vi "VI Quality.vi"() -> ()   [LabVIEW 2018, in "VI Quality.lvlib"]
doc: "This is the top level VI for the VI Quality Assurance user interface."
uses:
  VI Quality.lvlib
  <vilib>/LabVIEW Icon API/LabVIEW Icon API.lvlib
  <vilib>/Utility/miscctls.llb/LVRowAndColumnUnsignedTypeDef.ctl
  <vilib>/Utility/miscctls.llb/LVPointTypeDef.ctl
  <vilib>/Utility/miscctls.llb/LVSelectionTypeDef.ctl
  <vilib>/LabVIEW Icon API/lv_icon/Classes/Icon/Icon.lvclass
  Controls/VIQA VI Info.ctl
  Controls/VIQA Audit Ignore.ctl
panel:
  in  "Fix All":bool
  in  "ResetVI":bool
  out "VIBusy":bool
  in  "Edit Icon":bool
  in  "Reset Legal":bool
  in  "Legal":string caption="Legal Marking"
  out "VI Name":string
  in  "Ignore":T1
  in  "Abort":bool
  out "BusyAud":bool
  out "AuditSlide":dbl(slide) scale=0.0..100.0
  in  "AuditMCLB":i32(listbox) caption="Audit"
  in  "Audit":bool
  out "Busy":bool
  in  "Filter":enum16{"None", "No Description"}(ring)
  in  "Path Refresh":bool
  in  "Apply":bool
  in  "VI Description":string
  out "VI Path":path
  in  "Stop":bool
  out "ConPane":picture caption="VI Icon"
  in  "Project Tree":string[](tree)
  in  "Path":path caption="Path (*.lvproj)"
  # "Audit"
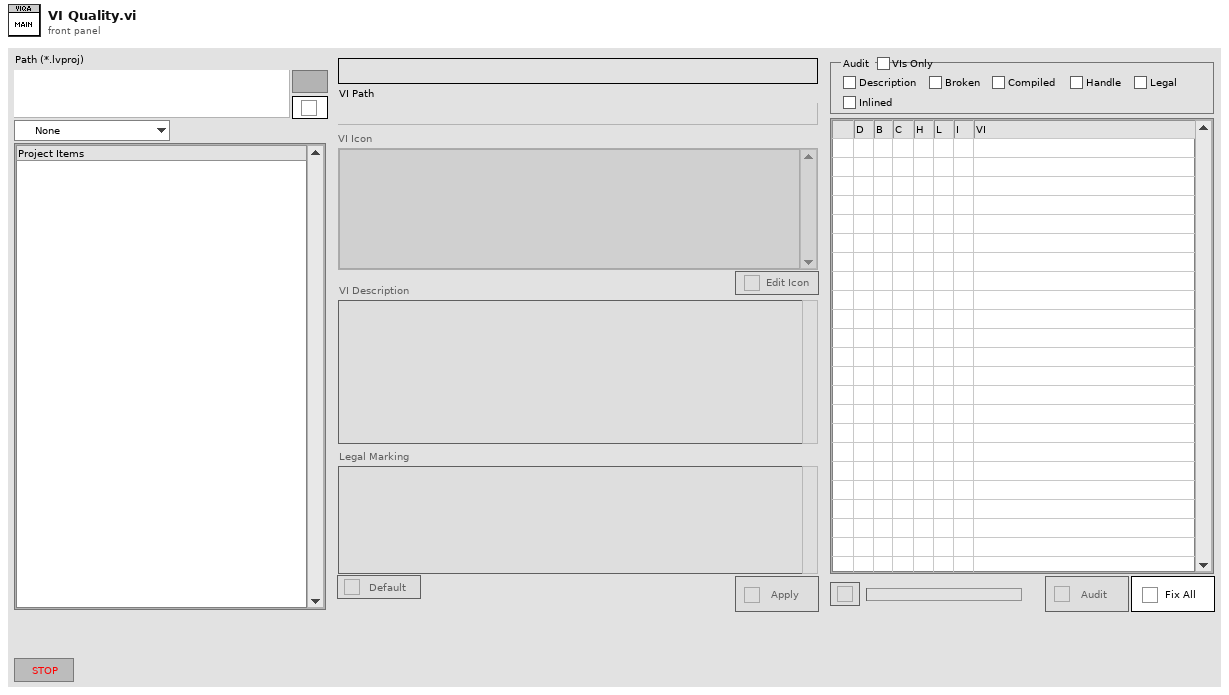
[diagram p1: front panel]
types:
  T1 = cluster{"Controls":bool, "Description":bool, "Broken":bool, "Compiled":bool, "Handle":bool, "Legal":bool, "Inlined":bool}
  T2 = cluster{"image type":i32, "image depth":i32, "image":u8[], "mask":u8[], "colors":u32[], "Rectangle":cluster{"left":i16, "top":i16, "right":i16, "bottom":i16}}[]
  T3 = typedef "VI Quality.lvlib/VIQA VI Info.ctl" = cluster{"Path":path, "Desc":string, "ConPane":cluster{"image type":i32, "image depth":i32, "image":u8[], "mask":u8[], "colors":u32[], "Rectangle":cluster{"left":i16, "top":i16, "right":i16, "bottom":i16}}, "Legal":string, "Icon":refnum<class "Icon.lvclass">, "VIType":enum32{"invalid VI type", "Standard VI", "Control VI", "Global VI", "Polymorphic VI", "Configuration VI", "SubSystem", "Facade VI", "Method VI", "Statechart Diagram VI"}, "ItemID":string}
  T4 = cluster{"Project Tree":refnum<vi>, "App Ref":refnum<vi>, "Project":refnum<vi>, "My Computer":refnum<vi>, "VI Refnum":refnum<vi>, "VI Info":T3, "AuditMCLB":refnum<vi>, "AuditSlide":refnum<vi>, "NewDesc":string, "NewLegal":string, "NewIcon":bool, "Abort":refnum<vi>}
  T5 = typedef "LVRowAndColumnUnsignedTypeDef.ctl" = cluster{"Row":u32, "Column":u32}
  T6 = typedef "VI Quality.lvlib/VIQA Audit Ignore.ctl" = cluster{"Controls":bool, "Description":bool, "Broken":bool, "Compiled":bool, "Handle":bool, "Legal":bool, "Inline":bool}
  T7 = typedef "LVPointTypeDef.ctl" = cluster{"Horizontal":i16, "Vertical":i16}
  T8 = typedef "LVSelectionTypeDef.ctl" = cluster{"Selection Start":u32, "Selection End":u32}
  T9 = cluster{"image type":i32, "image depth":i32, "image":u8[], "mask":u8[], "colors":u32[], "Rectangle":cluster{"left":i16, "top":i16, "right":i16, "bottom":i16}}
  T10 = enum32{"invalid VI type", "Standard VI", "Control VI", "Global VI", "Polymorphic VI", "Configuration VI", "SubSystem", "Facade VI", "Method VI", "Statechart Diagram VI"}
  T11 = enum8{"Enabled", "Disabled", "Disabled and Grayed Out"}
  T12 = typedef "imagedata.ctl" = cluster{"image type":i32, "image depth":i32, "image":u8[], "mask":u8[], "colors":u32[], "Rectangle":cluster{"left":i16, "top":i16, "right":i16, "bottom":i16}}
  T13 = cluster{"Shift":bool, "Ctrl":bool, "Alt":bool, "Cmd":bool, "Opt":bool}
  T14 = typedef "eventvkey.ctl" = enum16{"ASCII", "Enter", "Return", "Shift", "Ctrl", "Alt", "Cmd", "Opt", "Caps", "NumLock", "Clear", "Break", "Up", "Down", "Left", "Right", "Insert", "Delete", "Home", "End", "PageUp", "PageDown", "Escape", "Help", "Pause", "ScrollLock", "F1", "F2", "F3", "F4", "F5", "F6", "F7", "F8", "F9", "F10", "F11", "F12", "F13", "F14", "F15", "F16", "F17", "F18", "F19", "F20", "F21", "F22", "F23", "F24", "Play", "VolumeUp", "VolumeDown", "Mute", "Two Byte Char"}
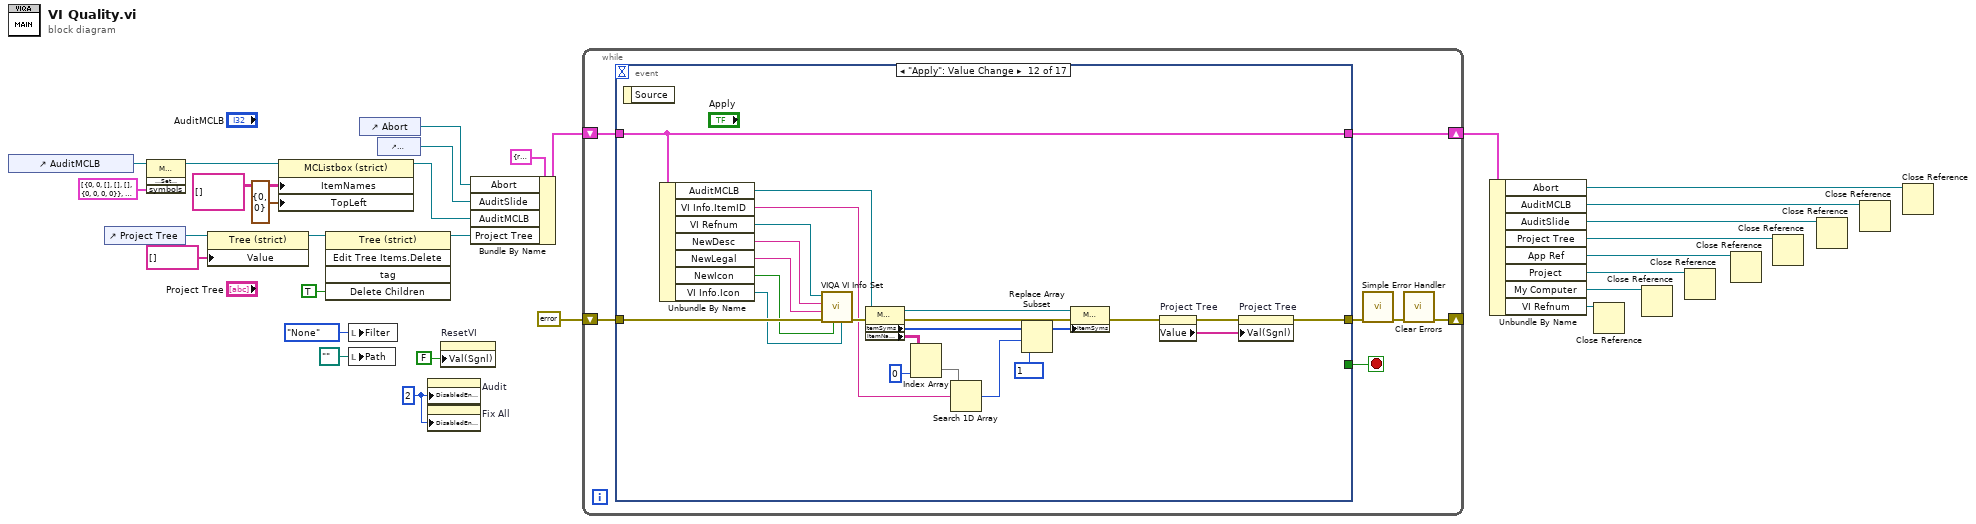
[diagram p0: block diagram]
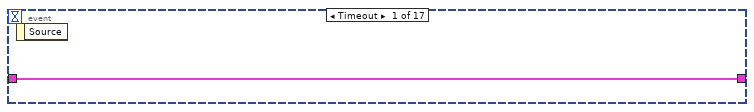
[diagram p2: hidden frame]
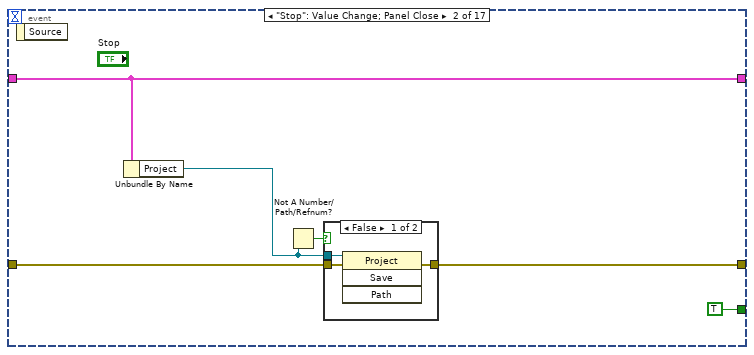
[diagram p3: hidden frame]
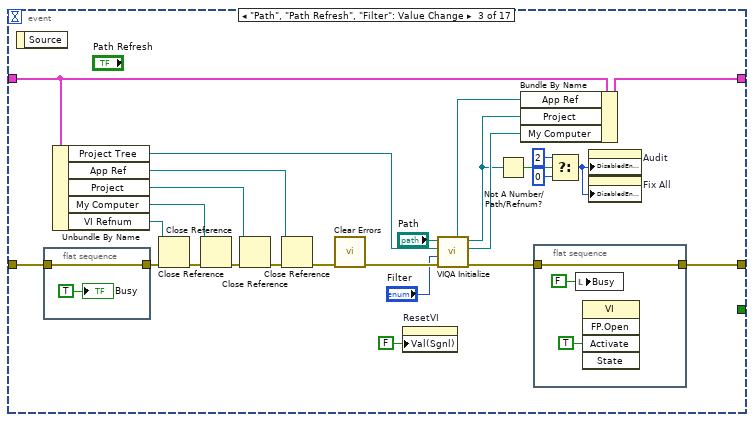
[diagram p5: hidden frame]
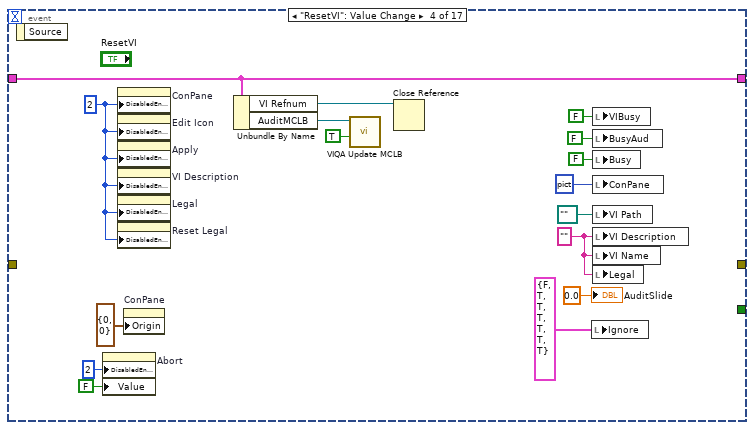
[diagram p6: hidden frame]
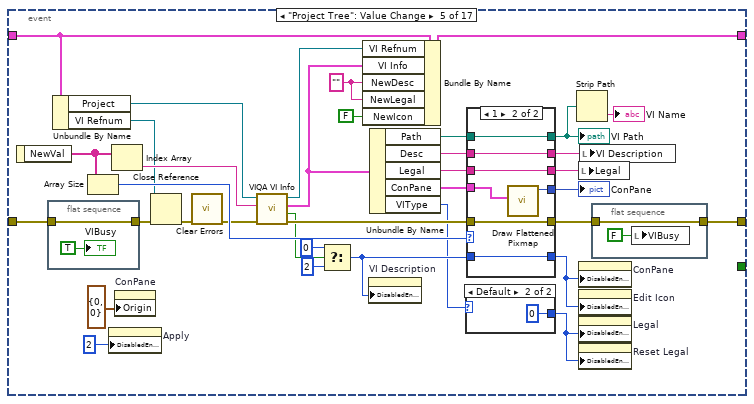
[diagram p7: hidden frame]
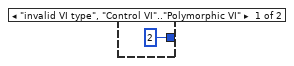
[diagram p8: hidden frame]
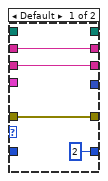
[diagram p9: hidden frame]
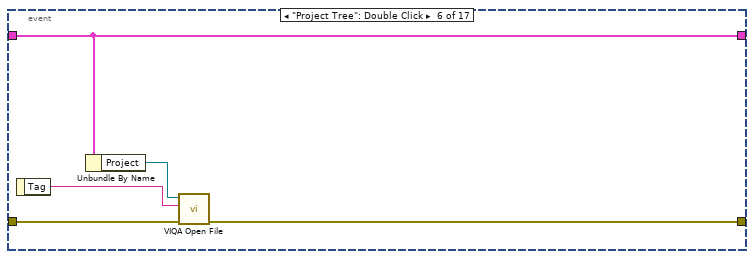
[diagram p10: hidden frame]
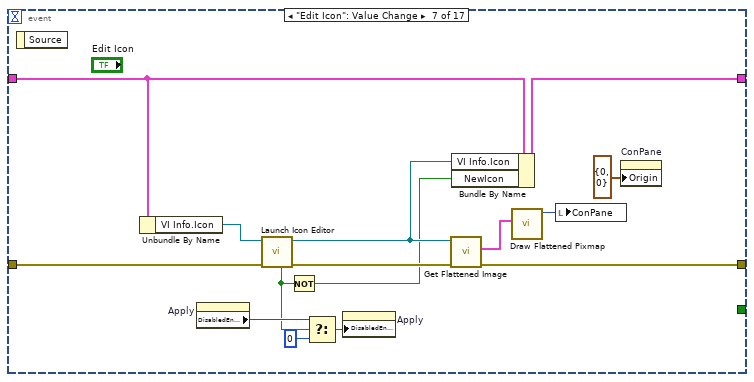
[diagram p11: hidden frame]
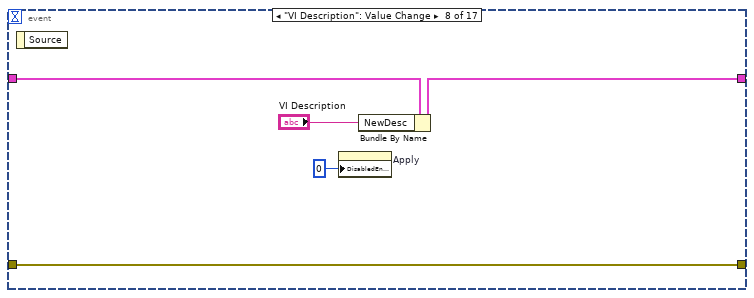
[diagram p12: hidden frame]
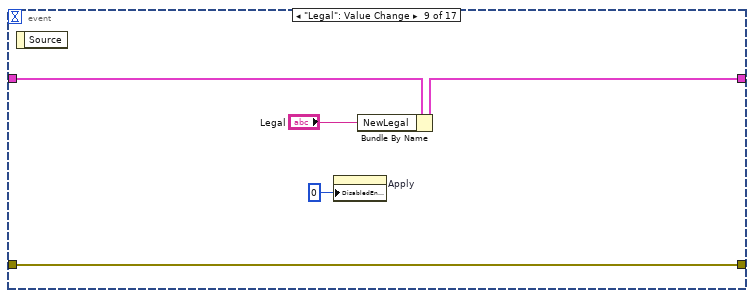
[diagram p13: hidden frame]
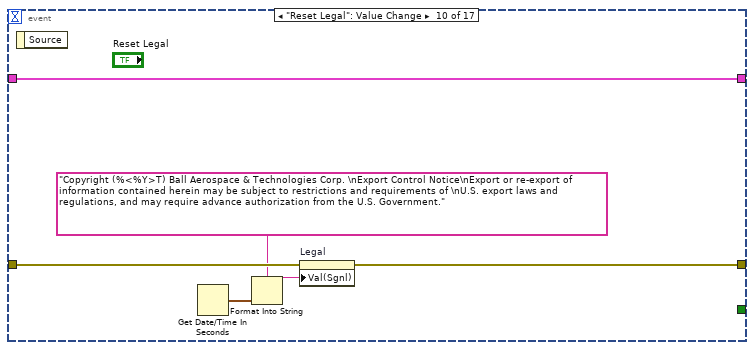
[diagram p14: hidden frame]
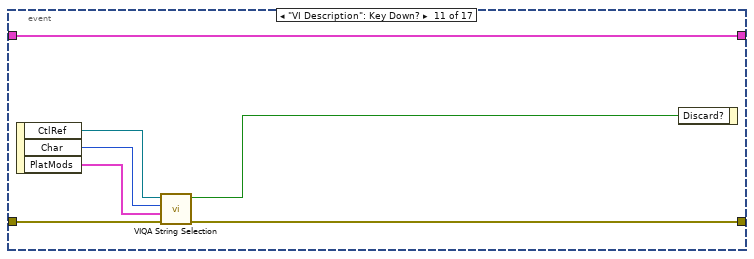
[diagram p15: hidden frame]
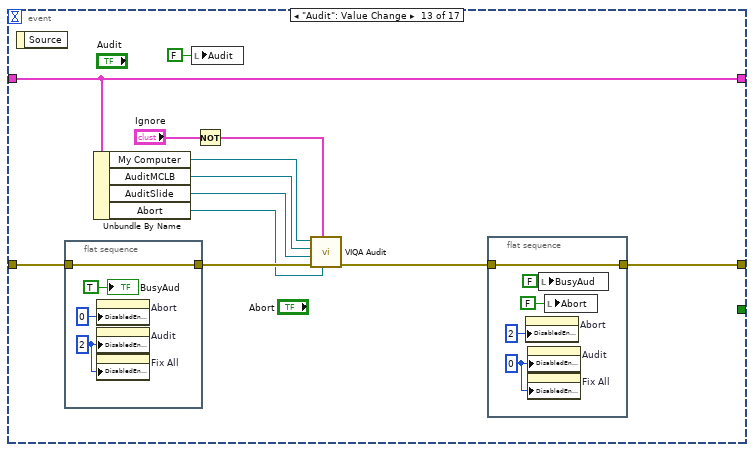
[diagram p16: hidden frame]
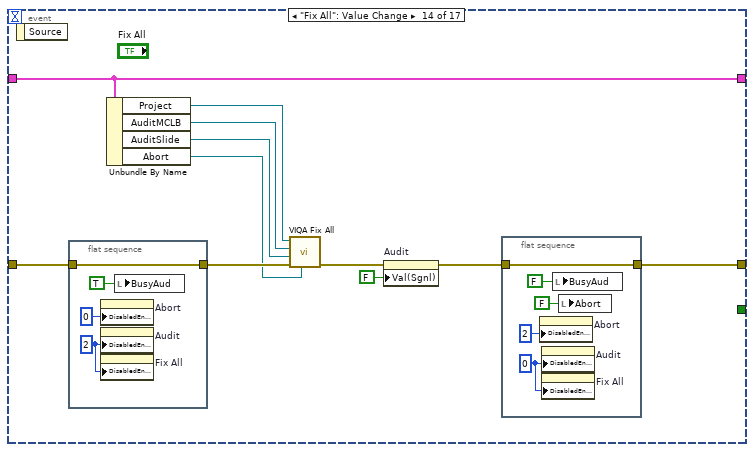
[diagram p17: hidden frame]
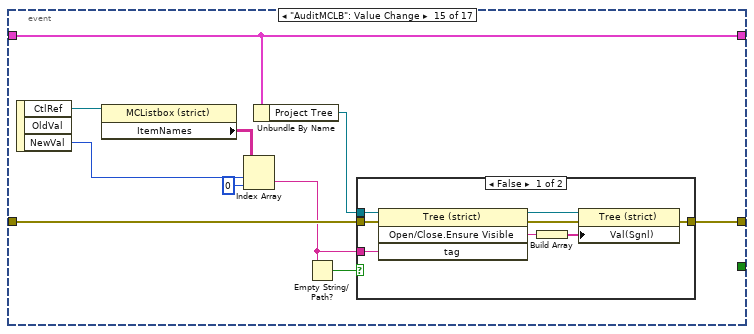
[diagram p18: hidden frame]
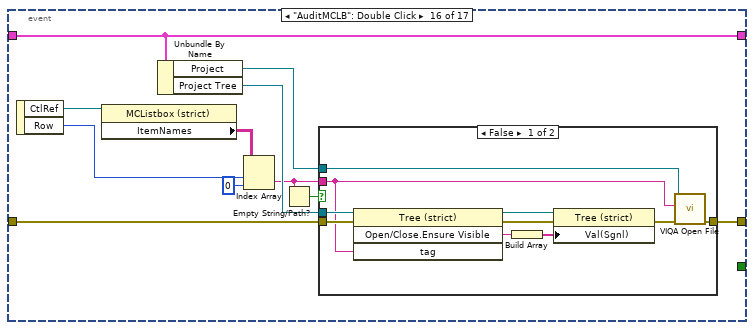
[diagram p20: hidden frame]
diagram:
  w5 = u8 2
  n1 = control-ref of="AuditMCLB"() -> (w15:refnum<vi>)
  n2 = control-ref of="Project Tree"() -> (w26:refnum<vi>)
  n3 = invoke class="MCListbox (strict)" method="Custom Item Symbols.Set Symbol Array"(reference=w15, "symbols"=T2 [{"image type"=0, "image depth"=0, "image"=[], "mask"=[], "colors"=[], "Rectangle"={"left"=0, "top"=0, "right"=0, "bottom"=0}}, {"image type"=0, "image depth"=32, "image"=[0, 0, 0, 0, 0, 0, 0, 0, 0, 0, 0, 0, 0, 0, 0, 0, 0, 0, 0, 0, 0, 0, 0, 0, 0, 0, 0, 0, 0, 0, 0, 0, 0, 0, 0, 0, 0, 0, 0, 0, 0, 0, 0, 0, 0, 0, 0, 0, 0, 0, 0, 0, 0, 0, 0, 0, 0, 0, 0, 0, 0, 0, 0, 0, 0, 0, 0, 0, 0, 0, 0, 0, 0, 0, 0, 0, 0, 0, 0, 0, 0, 0, 0, 0, 0, 0, 0, 0, 0, 0, 0, 0, 0, 0, 0, 0, 0, 0, 0, 0, 0, 0, 0, 0, 0, 0, 0, 0, 0, 0, 0, 0, 0, 0, 0, 0, 0, 0, 0, 0, 0, 0, 0, 0, 0, 0, 0, 0, 0, 0, 0, 0, 0, 0, 0, 0, 0, 0, 0, 0, 0, 0, 0, 0, 0, 0, 0, 0, 0, 0, 0, 0, 0, 0, 0, 0, 0, 0, 0, 0, 0, 0, 0, 0, 0, 0, 0, 0, 0, 0, 0, 0, 0, 0, 0, 0, 0, 0, 0, 0, 0, 0, 0, 0, 255, 133, 241, 88, 255, 85, 205, 56, 0, 0, 0, 0, 0, 0, 0, 0, 0, 0, 0, 0, 0, 0, 0, 0, 0, 0, 0, 0, 0, 0, 0, 0, 0, 0, 0, 0, 0, 0, 0, 0, 0, 0, 0, 0, 0, 0, 0, 0, 0, 0, 0, 0, 0, 0, 0, 0, 255, 121, 232, 80, 255, 121, 232, 80, 255, 121, 232, 80, 255, 85, 205, 56, 0, 0, 0, 0, 0, 0, 0, 0, 0, 0, 0, 0, 0, 0, 0, 0, 0, 0, 0, 0, 0, 0, 0, 0, 0, 0, 0, 0, 0, 0, 0, 0, 0, 0, 0, 0, 0, 0, 0, 0, 0, 0, 0, 0, 255, 109, 223, 72, 255, 109, 223, 72, 255, 109, 223, 72, 255, 109, 223, 72, 255, 0, 141, 0, 0, 0, 0, 0, 0, 0, 0, 0, 0, 0, 0, 0, 0, 0, 0, 0, 0, 0, 0, 0, 0, 0, 0, 0, 0, 0, 0, 0, 0, 0, 0, 0, 0, 0, 0, 0, 0, 0, 0, 0, 255, 97, 214, 64, 255, 97, 214, 64, 255, 97, 214, 64, 255, 97, 214, 64, 255, 0, 141, 0, 0, 0, 0, 0, 0, 0, 0, 0, 0, 0, 0, 0, 0, 0, 0, 0, 0, 0, 0, 0, 0, 0, 0, 0, 0, 0, 0, 0, 0, 0, 0, 0, 0, 0, 0, 0, 0, 0, 0, 0, 255, 85, 205, 56, 255, 85, 205, 56, 255, 85, 205, 56, 255, 85, 205, 56, 255, 0, 141, 0, 0, 0, 0, 0, 0, 0, 0, 0, 0, 0, 0, 0, 255, 73, 196, 48, 255, 73, 196, 48, 255, 73, 196, 48, 0, 0, 0, 0, 0, 0, 0, 0, 0, 0, 0, 0, 0, 0, 0, 0, 255, 73, 196, 48, 255, 73, 196, 48, 255, 73, 196, 48, 255, 73, 196, 48, 255, 0, 141, 0, 0, 0, 0, 0, 0, 0, 0, 0, 0, 0, 0, 0, 0, 0, 0, 0, 255, 12, 150, 8, 255, 60, 186, 40, 255, 60, 186, 40, 255, 60, 186, 40, 0, 0, 0, 0, 0, 0, 0, 0, 255, 60, 186, 40, 255, 60, 186, 40, 255, 60, 186, 40, 255, 60, 186, 40, 255, 0, 141, 0, 0, 0, 0, 0, 0, 0, 0, 0, 0, 0, 0, 0, 0, 0, 0, 0, 0, 0, 0, 0, 255, 0, 141, 0, 255, 48, 177, 32, 255, 48, 177, 32, 255, 48, 177, 32, 255, 48, 177, 32, 255, 48, 177, 32, 255, 48, 177, 32, 255, 48, 177, 32, 255, 48, 177, 32, 255, 0, 141, 0, 0, 0, 0, 0, 0, 0, 0, 0, 0, 0, 0, 0, 0, 0, 0, 0, 0, 0, 0, 0, 0, 0, 0, 0, 0, 0, 0, 0, 255, 0, 141, 0, 255, 36, 168, 24, 255, 36, 168, 24, 255, 36, 168, 24, 255, 36, 168, 24, 255, 36, 168, 24, 255, 36, 168, 24, 255, 0, 141, 0, 0, 0, 0, 0, 0, 0, 0, 0, 0, 0, 0, 0, 0, 0, 0, 0, 0, 0, 0, 0, 0, 0, 0, 0, 0, 0, 0, 0, 0, 0, 0, 0, 0, 0, 0, 0, 255, 0, 141, 0, 255, 24, 159, 16, 255, 24, 159, 16, 255, 24, 159, 16, 255, 24, 159, 16, 255, 0, 141, 0, 0, 0, 0, 0, 0, 0, 0, 0, 0, 0, 0, 0, 0, 0, 0, 0, 0, 0, 0, 0, 0, 0, 0, 0, 0, 0, 0, 0, 0, 0, 0, 0, 0, 0, 0, 0, 0, 0, 0, 0, 0, 0, 0, 0, 255, 0, 141, 0, 255, 12, 150, 8, 255, 12, 150, 8, 255, 0, 141, 0, 0, 0, 0, 0, 0, 0, 0, 0, 0, 0, 0, 0, 0, 0, 0, 0, 0, 0, 0, 0, 0, 0, 0, 0, 0, 0, 0, 0, 0, 0, 0, 0, 0, 0, 0, 0, 0, 0, 0, 0, 0, 0, 0, 0, 0, 0, 0, 0, 0, 0, 0, 0, 255, 0, 141, 0, 255, 0, 141, 0, 0, 0, 0, 0, 0, 0, 0, 0, 0, 0, 0, 0, 0, 0, 0, 0, 0, 0, 0, 0, 0, 0, 0, 0, 0, 0, 0, 0, 0, 0, 0, 0, 0, 0, 0, 0, 0, 0, 0, 0, 0, 0, 0, 0, 0, 0, 0, 0, 0, 0, 0, 0, 0, 0, 0, 0, 0, 0, 0, 0, 0, 0, 0, 0, 0, 0, 0, 0, 0, 0, 0, 0, 0, 0, 0, 0, 0, 0, 0, 0, 0, 0, 0, 0, 0, 0, 0, 0, 0, 0, 0, 0, 0, 0, 0, 0, 0, 0, 0, 0, 0, 0, 0, 0, 0, 0, 0, 0, 0, 0, 0, 0, 0, 0, 0, 0, 0, 0, 0, 0, 0, 0, 0, 0, 0, 0, 0, 0, 0, 0, 0, 0, 0, 0, 0, 0, 0, 0, 0, 0, 0, 0, 0, 0, 0, 0, 0, 0, 0, 0, 0, 0, 0, 0, 0, 0, 0, 0, 0, 0, 0, 0, 0, 0], "mask"=[0, 0, 0, 0, 0, 3, 0, 15, 0, 31, 0, 62, 0, 124, 112, 248, 121, 240, 127, 224, 63, 192, 31, 128, 15, 0, 6, 0, 0, 0, 0, 0], "colors"=[], "Rectangle"={"left"=0, "top"=0, "right"=16, "bottom"=16}}] ("Symbols")) -> (reference out=w2:refnum<vi>)  [unwired: 2 in, 3 out]
  n4 = property class="Tree (strict)"(reference=w26, "Value"=string[] []) -> (reference out=w18:refnum<vi>)  [unwired: 1 in, 1 out]
  n5 = property class="MCListbox (strict)"(reference=w2, "ItemNames"=string[][] [] ("Item Names"), "TopLeft"=T5 {"Row"=0, "Column"=0} ("Top Left Visible Cell")) -> (reference out=w13:refnum<vi>)  [unwired: 1 in, 1 out]
  n6 = invoke class="Tree (strict)" method="Edit Tree Items.Delete"(reference=w18, "Delete Children"=TRUE ("Delete Children?")) -> (reference out=w25:refnum<vi>)  [unwired: 3 in, 4 out]
  n7 = local write "Filter"(enum16{"None", "No Description", "No Legend"}."None" ("Filter")) -> ()
  n8 = local write "Path"(path "" ("Path")) -> ()
  n9 = control-ref of="Abort"() -> (w4:refnum<vi>)
  n10 = control-ref of="AuditSlide"() -> (w14:refnum<vi>)
  n11 = property on="Audit" class="Bool (strict)"("DisabledEnum"=w5) -> ()  [unwired: 2 in, 2 out]
  n12 = property on="Fix All" class="Bool"("DisabledEnum"=w5) -> ()  [unwired: 2 in, 2 out]
  n13 = property on="ResetVI" class="Bool (strict)"("Val(Sgnl)"=FALSE ("Value (Signaling)")) -> ()  [unwired: 2 in, 2 out]
  n14 = Bundle By Name(cluster=T4 {"Project Tree"=refnum, "App Ref"=refnum, "Project"=refnum, "My Computer"=refnum, "VI Refnum"=refnum, "VI Info"={"Path"=path "", "Desc"="", "ConPane"={"image type"=0, "image depth"=0, "image"=[], "mask"=[], "colors"=[], "Rectangle"={"left"=0, "top"=0, "right"=0, "bottom"=0}}, "Legal"="", "Icon"=refnum, "VIType"=enum."invalid VI type", "ItemID"=""}, "AuditMCLB"=refnum, "AuditSlide"=refnum, "NewDesc"="", "NewLegal"="", "NewIcon"=FALSE, "Abort"=refnum} ("StateData"), "Abort"=w4, "AuditSlide"=w14, "AuditMCLB"=w13, "Project Tree"=w25) -> (w27:T4)
  n15 = while {
    shift-right: [w30] -> _
    shift-left: errorcluster {"status"=FALSE, "code"=0, "source"=""} ("error in (no error)") -> [w35]
    shift-right: [w32] -> w23
    shift-left: w27 -> [w33]
    stop <- w36 stop-if-true
    n16 = event shown="[11] \"Apply\": Value Change" {
      selector: _ -> [_ _ _ _ _ _ _ _ _ _ _ _ _ _ _ _ _]
      dyn-events: _ -> [_ _ _ _ _ _ _ _ _ _ _ _ _ _ _ _ _]
      timeout: _ -> [_ _ _ _ _ _ _ _ _ _ _ _ _ _ _ _ _]
      tunnel: [_ TRUE _ _ _ _ _ _ _ _ _ _ _ _ _ _ _] -> w36
      tunnel: w35 -> [_ w42 w56 _ w97 w152 w164 w169 w174 w182 w188 w212 w221 w241 w259 w278 w298]
      tunnel: [_ w41 w55 _ w96 w149 w161 w169 w174 w181 w187 w205 w220 w242 w258 w277 w299] -> w34
      tunnel: w33 -> [w37 w40 w72 w82 w130 w151 w167 w172 w177 w183 w190 w213 w225 w245 w261 w280 w302]
      tunnel: [w37 w40 w65 w82 w127 w151 w166 w171 w176 w183 w190 w213 w225 w245 w261 w280 w302] -> w32
      event Timeout {
        n17 = event-data() -> ()  [unwired: 1 in, 1 out]
      }
      event "Stop": Value Change; Panel Close {
        n18 = event-data() -> ()  [unwired: 1 in, 1 out]
        n19 = Unbundle By Name(w40) -> ("Project"=w39:refnum<vi>)
        n20 = Not A Number/Path/Refnum?(number/path/refnum=w39) -> (NaN/Path/Refnum?=w38:bool)
        n21 = case shown="False" w38 {
          tunnel: w42 -> [w46 w47]
          tunnel: [w45 w47] -> w41
          tunnel: w39 -> [w44 _]
          frame False {
            n22 = invoke class="Project" method="Save"(reference=w44, error in=w46) -> (error out=w45:errorcluster)  [unwired: 2 in, 3 out]
          }
          frame True {
          }
        }
      }
      event "Path", "Path Refresh", "Filter": Value Change {
        n23 = event-data() -> ()  [unwired: 1 in, 1 out]
        n24 = flat-sequence {
          tunnel: [w77] -> w57
          tunnel: w56 -> [w77]
          frame #0 {
            "Busy" <- TRUE ("Loading")
          }
        }
        n25 = Unbundle By Name(w72) -> ("Project Tree"=w71:refnum<vi>, "App Ref"=w59:refnum<vi>, "Project"=w67:refnum<vi>, "My Computer"=w69:refnum<vi>, "VI Refnum"=w61:refnum<vi>)
        n26 = Close Reference(reference=w61, error in (no error)=w57) -> (error out=w62:errorcluster)
        n27 = Close Reference(reference=w69, error in (no error)=w62) -> (error out=w70:errorcluster)
        n28 = Close Reference(reference=w67, error in (no error)=w70) -> (error out=w68:errorcluster)
        n29 = Close Reference(reference=w59, error in (no error)=w68) -> (error out=w60:errorcluster)
        n30 = call <vilib>:"Clear Errors.vi"("error in (no error)"=w60) -> ("error out"=w66:errorcluster)  [unwired: 5 in, 1 out]
        n31 = property on="ResetVI" class="Bool (strict)"("Val(Sgnl)"=FALSE ("Value (Signaling)")) -> ()  [unwired: 2 in, 2 out]
        n32 = call "VIQA Initialize.vi"("error in (no error)"=w66, "Filter"="Filter", "Project Tree"=w71, "Project (*.lvproj)"="Path") -> ("error out"=w54:errorcluster, "My Computer"=w64:refnum<vi>, "Project"=w53:refnum<vi>, "App Ref"=w63:refnum<vi>)  [unwired: 4 in]
        n33 = Not A Number/Path/Refnum?(number/path/refnum=w53) -> (NaN/Path/Refnum?=w52:bool)
        n34 = Bundle By Name(cluster=w72, "App Ref"=w63, "Project"=w53, "My Computer"=w64) -> (w65:T4)
        n35 = flat-sequence {
          tunnel: [w75] -> w55
          tunnel: w54 -> [w75]
          frame #0 {
            n36 = local write "Busy"(FALSE ("Busy")) -> ()
            n37 = invoke class="VI" method="FP.Open"("Activate"=TRUE ("Activate?")) -> ()  [unwired: 4 in, 5 out]
          }
        }
        n38 = Select(t=u8 2, s=w52, f=u8 0) -> (s? t:f=w48:u8)
        n39 = property on="Audit" class="Bool (strict)"("DisabledEnum"=w48) -> ()  [unwired: 2 in, 2 out]
        n40 = property on="Fix All" class="Bool"("DisabledEnum"=w48) -> ()  [unwired: 2 in, 2 out]
      }
      event "ResetVI": Value Change {
        w84 = "" ("VI Description")
        w94 = u8 2
        n41 = event-data() -> ()  [unwired: 1 in, 1 out]
        n42 = property on="Abort" class="Bool (strict)"("DisabledEnum"=u8 2, "Value"=FALSE ("Abort")) -> ()  [unwired: 2 in, 2 out]
        n43 = property on="ConPane" class="Pict"("DisabledEnum"=w94) -> ()  [unwired: 2 in, 2 out]
        n44 = property on="Edit Icon" class="Bool"("DisabledEnum"=w94) -> ()  [unwired: 2 in, 2 out]
        n45 = property on="Apply" class="Bool"("DisabledEnum"=w94) -> ()  [unwired: 2 in, 2 out]
        n46 = property on="VI Description" class="Str"("DisabledEnum"=w94) -> ()  [unwired: 2 in, 2 out]
        n47 = property on="Legal" class="Str"("DisabledEnum"=w94) -> ()  [unwired: 2 in, 2 out]
        n48 = property on="Reset Legal" class="Bool"("DisabledEnum"=w94) -> ()  [unwired: 2 in, 2 out]
        n49 = property on="ConPane" class="Pict"("Origin"=T7 {"Horizontal"=0, "Vertical"=0}) -> ()  [unwired: 2 in, 2 out]
        n50 = Unbundle By Name(w82) -> ("VI Refnum"=w80:refnum<vi>, "AuditMCLB"=w81:refnum<vi>)
        n51 = call "VIQA Update MCLB.vi"("Reset TopLeft? (F)"=TRUE, "MCLB"=w81) -> ()  [unwired: 8 in, 2 out]
        n52 = Close Reference(reference=w80) -> ()  [unwired: 1 in, 1 out]
        n53 = local write "Ignore"(T6 {"Controls"=FALSE, "Description"=TRUE, "Broken"=TRUE, "Compiled"=TRUE, "Handle"=TRUE, "Legal"=TRUE, "Inline"=TRUE} ("Ignore")) -> ()
        n54 = local write "VIBusy"(FALSE ("VIBusy")) -> ()
        n55 = local write "BusyAud"(FALSE ("Busy2")) -> ()
        n56 = local write "Busy"(FALSE ("Busy")) -> ()
        n57 = local write "ConPane"(picture data[5B] ("picture")) -> ()
        n58 = local write "VI Path"(path "" ("VI Path")) -> ()
        n59 = local write "VI Description"(w84) -> ()
        n60 = local write "VI Name"(w84) -> ()
        n61 = local write "Legal"(w84) -> ()
        "AuditSlide" <- 0.0 ("AuditStatus")
      }
      event "Project Tree": Value Change {
        w100 = "" ("NewDesc")
        n62 = event-data() -> ("NewVal"=w125:string[])  [unwired: 1 in]
        n63 = flat-sequence {
          tunnel: [w133] -> w98
          tunnel: w97 -> [w133]
          frame #0 {
            "VIBusy" <- TRUE ("VIBusy")
          }
        }
        n64 = Unbundle By Name(w130) -> ("Project"=w128:refnum<vi>, "VI Refnum"=w114:refnum<vi>)
        n65 = Array Size(array=w125) -> (size(s)=w124:i32)
        n66 = property on="Apply" class="Bool"("DisabledEnum"=u8 2) -> ()  [unwired: 2 in, 2 out]
        n67 = Index Array(array=w125) -> (element=w129:string)  [unwired: 1 in]
        n68 = property on="ConPane" class="Pict"("Origin"=T7 {"Horizontal"=0, "Vertical"=0}) -> ()  [unwired: 2 in, 2 out]
        n69 = Close Reference(reference=w114, error in (no error)=w98) -> (error out=w115:errorcluster)
        n70 = call <vilib>:"Clear Errors.vi"("error in (no error)"=w115) -> ("error out"=w113:errorcluster)  [unwired: 5 in, 1 out]
        n71 = call "VIQA VI Info.vi"("error in (no error)"=w113, "Item ID"=w129, "Project"=w128) -> ("error out"=w121:errorcluster, "Valid?"=w105:bool, "VI Info"=w126:T3, "VI Refnum"=w112:refnum<vi>)  [unwired: 5 in]
        n72 = Select(t=u8 0, s=w105, f=u8 2) -> (s? t:f=w104:u8)
        n73 = Bundle By Name(cluster=w130, "VI Refnum"=w112, "VI Info"=w126, "NewDesc"=w100, "NewLegal"=w100, "NewIcon"=FALSE) -> (w127:T4)
        n74 = property on="VI Description" class="Str"("DisabledEnum"=w104) -> ()  [unwired: 2 in, 2 out]
        n75 = Unbundle By Name(w126) -> ("Path"=w120:path, "Desc"=w119:string, "Legal"=w108:string, "ConPane"=w122:T9, "VIType"=w102:T10)
        n76 = case shown="Default" w102 {
          tunnel: [u8 2 u8 0] -> w101
          frame "invalid VI type", "Control VI".."Polymorphic VI" {
          }
          frame Default {
          }
        }
        n77 = case shown="1" w124 {
          tunnel: [u8 2 w142] -> w106
          tunnel: [_ w147] -> w123
          tunnel: w122 -> [_ w146]
          tunnel: [w140 w145] -> w95
          tunnel: w121 -> [w140 w145]
          tunnel: [_ w144] -> w110
          tunnel: w120 -> [_ w144]
          tunnel: w119 -> [w139 w143]
          tunnel: [w139 w143] -> w116
          tunnel: w104 -> [_ w142]
          tunnel: [w137 w141] -> w107
          tunnel: w108 -> [w137 w141]
          frame Default {
          }
          frame 1 {
            n78 = call <vilib>:"Draw Flattened Pixmap.vi"("image data"=w146) -> ("new picture"=w147:picture)  [unwired: 8 in]
          }
        }
        "VI Path" <- w110
        "ConPane" <- w123
        n79 = Strip Path(path=w110) -> (name=→"VI Name":string)  [unwired: 1 out]
        n80 = local write "Legal"(w107) -> ()
        n81 = property on="ConPane" class="Pict"("DisabledEnum"=w106) -> ()  [unwired: 2 in, 2 out]
        n82 = property on="Edit Icon" class="Bool"("DisabledEnum"=w106) -> ()  [unwired: 2 in, 2 out]
        n83 = property on="Legal" class="Str"("DisabledEnum"=w101) -> ()  [unwired: 2 in, 2 out]
        n84 = property on="Reset Legal" class="Bool"("DisabledEnum"=w101) -> ()  [unwired: 2 in, 2 out]
        n85 = local write "VI Description"(w116) -> ()
        n86 = flat-sequence {
          tunnel: [w131] -> w96
          tunnel: w95 -> [w131]
          frame #0 {
            n87 = local write "VIBusy"(FALSE ("VIBusy")) -> ()
          }
        }
      }
      event "Project Tree": Double Click {
        n88 = event-data() -> ("Tag"=w150:string)  [unwired: 1 in]
        n89 = Unbundle By Name(w151) -> ("Project"=w148:refnum<vi>)
        n90 = call "VIQA Open File.vi"("error in (no error)"=w152, "Tag"=w150, "Project in"=w148) -> ("error out"=w149:errorcluster)  [unwired: 8 in]
      }
      event "Edit Icon": Value Change {
        n91 = event-data() -> ()  [unwired: 1 in, 1 out]
        n92 = Unbundle By Name(w167) -> ("VI Info.Icon"=w163:refnum<class "Icon.lvclass">)
        n93 = property on="Apply" class="Bool"() -> ("DisabledEnum"=w157:T11)  [unwired: 2 in, 2 out]
        n94 = call <vilib>:"Launch Icon Editor.vi"("error in (no error)"=w164, "Icon in"=w163) -> ("error out"=w162:errorcluster, "Icon out"=w160:refnum<class "Icon.lvclass">, "Canceled?"=w154:bool)  [unwired: 7 in]
        n95 = Not(x=w154) -> (.not. x?=w153:bool)
        n96 = Select(t=w157, s=w154, f=u8 0) -> (s? t:f=w155:u8)
        n97 = property on="Apply" class="Bool"("DisabledEnum"=w155) -> ()  [unwired: 2 in, 2 out]
        n98 = call <vilib>:"Get Flattened Image.vi"("error in (no error)"=w162, "lv_icon.lvlib:Icon.lvclass in"=w160) -> ("error out"=w161:errorcluster, "Color Image"=w159:T12)  [unwired: 6 in, 2 out]
        n99 = Bundle By Name(cluster=w167, "VI Info.Icon"=w160, "NewIcon"=w153) -> (w166:T4)
        n100 = call <vilib>:"Draw Flattened Pixmap.vi"("image data"=w159) -> ("new picture"=w165:picture)  [unwired: 8 in]
        n101 = local write "ConPane"(w165) -> ()
        n102 = property on="ConPane" class="Pict"("Origin"=T7 {"Horizontal"=0, "Vertical"=0}) -> ()  [unwired: 2 in, 2 out]
      }
      event "VI Description": Value Change {
        n103 = event-data() -> ()  [unwired: 1 in, 1 out]
        n104 = property on="Apply" class="Bool"("DisabledEnum"=u8 0) -> ()  [unwired: 2 in, 2 out]
        n105 = Bundle By Name(cluster=w172, "NewDesc"="VI Description") -> (w171:T4)
      }
      event "Legal": Value Change {
        n106 = event-data() -> ()  [unwired: 1 in, 1 out]
        n107 = property on="Apply" class="Bool"("DisabledEnum"=u8 0) -> ()  [unwired: 2 in, 2 out]
        n108 = Bundle By Name(cluster=w177, "NewLegal"="Legal") -> (w176:T4)
      }
      event "Reset Legal": Value Change {
        n109 = event-data() -> ()  [unwired: 1 in, 1 out]
        n110 = Get Date/Time In Seconds() -> (seconds since 1Jan1904=w178:timestamp)
        n111 = Format Into String(format string="Copyright (%<%Y>T) Ball Aerospace & Technologies Corp. \nExport Control Notice\nExport or re-export of information contained herein may be subject to restrictions and requirements of \nU.S. export laws and regulations, and may require advance authorization from the U.S. Government.", w178) -> (resulting string=w179:string)  [unwired: 2 in, 1 out]
        n112 = property on="Legal" class="Str"(error in=w182, "Val(Sgnl)"=w179) -> (error out=w181:errorcluster)  [unwired: 1 in, 1 out]
      }
      event "VI Description": Key Down? {
        n113 = event-data() -> ("CtlRef"=w189:refnum<vi>, "Char"=w186:i16, "PlatMods"=w184:T13)  [unwired: 1 in]
        n114 = call "VIQA String Selection.vi"("error in (no error)"=w188, "PlatMods"=w184, "Char"=w186, "String in"=w189) -> ("error out"=w187:errorcluster, "Discard"=w185:bool)  [unwired: 6 in]
        n115 = event-data("Discard?"=w185) -> ()  [unwired: 1 in, 1 out]
      }
      event "Apply": Value Change {
        n116 = event-data() -> ()  [unwired: 1 in, 1 out]
        n117 = Unbundle By Name(w213) -> ("AuditMCLB"=w202:refnum<vi>, "VI Info.ItemID"=w196:string, "VI Refnum"=w204:refnum<vi>, "NewDesc"=w211:string, "NewLegal"=w210:string, "NewIcon"=w209:bool, "VI Info.Icon"=w208:refnum<class "Icon.lvclass">)
        n118 = call "VIQA VI Info Set.vi"("Icon"=w208, "NewIcon"=w209, "error in (no error)"=w212, "NewLegal"=w210, "NewDesc"=w211, "VI Refnum"=w204) -> ("error out"=w203:errorcluster)  [unwired: 4 in, 1 out]
        n119 = property class="MCListbox (strict)"(reference=w202, error in=w203) -> (reference out=w200:refnum<vi>, error out=w201:errorcluster, "ItemSyms"=w195:i32[], "ItemNames"=w199:string[][])
        n120 = Index Array(array=w199, index (col)=0 ("index (row)")) -> (element=w197:string[])  [unwired: 1 in]
        n121 = Search 1D Array(1D array=w197, element=w196) -> (index of element=w193:i32)  [unwired: 1 in]
        n122 = Replace Array Subset(array=w195, new element=1 ("Symbol"), index=w193) -> (w194:i32[])
        n123 = property class="MCListbox (strict)"(reference=w200, error in=w201, "ItemSyms"=w194) -> (error out=w198:errorcluster)  [unwired: 1 out]
        n124 = property on="Project Tree" class="Tree (strict)"(error in=w198) -> (error out=w207:errorcluster, "Value"=w206:string[])  [unwired: 1 in, 1 out]
        n125 = property on="Project Tree" class="Tree (strict)"(error in=w207, "Val(Sgnl)"=w206) -> (error out=w205:errorcluster)  [unwired: 1 in, 1 out]
      }
      event "Audit": Value Change {
        n126 = event-data() -> ()  [unwired: 1 in, 1 out]
        n127 = flat-sequence {
          tunnel: [w233] -> w222
          tunnel: w221 -> [w233]
          frame #0 {
            w231 = u8 2
            n128 = property on="Abort" class="Bool (strict)"("DisabledEnum"=u8 0) -> ()  [unwired: 2 in, 2 out]
            n129 = property on="Audit" class="Bool (strict)"("DisabledEnum"=w231) -> ()  [unwired: 2 in, 2 out]
            n130 = property on="Fix All" class="Bool"("DisabledEnum"=w231) -> ()  [unwired: 2 in, 2 out]
            "BusyAud" <- TRUE ("Busy2")
          }
        }
        n131 = Unbundle By Name(w225) -> ("My Computer"=w224:refnum<vi>, "AuditMCLB"=w223:refnum<vi>, "AuditSlide"=w218:refnum<vi>, "Abort"=w215:refnum<vi>)
        n132 = local write "Audit"(FALSE ("Audit")) -> ()
        n133 = Not(x="Ignore") -> (.not. x?=w217:T1)
        n134 = call "VIQA Audit.vi"("Abort"=w215, "Ignore"=w217, "error in (no error)"=w222, "AuditSlide"=w218, "AuditMCLB"=w223, "My Computer"=w224) -> ("error out"=w219:errorcluster)  [unwired: 4 in, 1 out]
        n135 = flat-sequence {
          tunnel: [w229] -> w220
          tunnel: w219 -> [w229]
          frame #0 {
            w226 = u8 0
            n136 = property on="Abort" class="Bool (strict)"("DisabledEnum"=u8 2) -> ()  [unwired: 2 in, 2 out]
            n137 = property on="Audit" class="Bool (strict)"("DisabledEnum"=w226) -> ()  [unwired: 2 in, 2 out]
            n138 = property on="Fix All" class="Bool"("DisabledEnum"=w226) -> ()  [unwired: 2 in, 2 out]
            n139 = local write "BusyAud"(FALSE ("Busy2")) -> ()
            n140 = local write "Abort"(FALSE ("Abort")) -> ()
          }
        }
      }
      event "Fix All": Value Change {
        n141 = event-data() -> ()  [unwired: 1 in, 1 out]
        n142 = flat-sequence {
          tunnel: [w249] -> w240
          tunnel: w241 -> [w249]
          frame #0 {
            w247 = u8 2
            n143 = property on="Abort" class="Bool (strict)"("DisabledEnum"=u8 0) -> ()  [unwired: 2 in, 2 out]
            n144 = property on="Audit" class="Bool (strict)"("DisabledEnum"=w247) -> ()  [unwired: 2 in, 2 out]
            n145 = property on="Fix All" class="Bool"("DisabledEnum"=w247) -> ()  [unwired: 2 in, 2 out]
            n146 = local write "BusyAud"(TRUE ("Busy2")) -> ()
          }
        }
        n147 = Unbundle By Name(w245) -> ("Project"=w244:refnum<vi>, "AuditMCLB"=w243:refnum<vi>, "AuditSlide"=w239:refnum<vi>, "Abort"=w238:refnum<vi>)
        n148 = call "VIQA Fix All.vi"("Abort"=w238, "error in (no error)"=w240, "Slide"=w239, "AuditMCLB"=w243, "Project in"=w244) -> ("error out"=w237:errorcluster)  [unwired: 6 in]
        n149 = property on="Audit" class="Bool (strict)"(error in=w237, "Val(Sgnl)"=FALSE ("Value (Signaling)")) -> (error out=w236:errorcluster)  [unwired: 1 in, 1 out]
        n150 = flat-sequence {
          tunnel: [w253] -> w242
          tunnel: w236 -> [w253]
          frame #0 {
            w250 = u8 0
            n151 = property on="Abort" class="Bool (strict)"("DisabledEnum"=u8 2) -> ()  [unwired: 2 in, 2 out]
            n152 = property on="Audit" class="Bool (strict)"("DisabledEnum"=w250) -> ()  [unwired: 2 in, 2 out]
            n153 = property on="Fix All" class="Bool"("DisabledEnum"=w250) -> ()  [unwired: 2 in, 2 out]
            n154 = local write "BusyAud"(FALSE ("Busy2")) -> ()
            n155 = local write "Abort"(FALSE ("Abort")) -> ()
          }
        }
      }
      event "AuditMCLB": Value Change {
        n156 = event-data() -> ("CtlRef"=w264:refnum<vi>, "NewVal"=w257:i32)  [unwired: 1 in, 1 out]
        n157 = property class="MCListbox (strict)"(reference=w264) -> ("ItemNames"=w263:string[][])  [unwired: 1 in, 2 out]
        n158 = Index Array(array=w263, index (row)=w257, index (col)=0 ("disabled index (col)")) -> (element=w256:string)
        n159 = Unbundle By Name(w261) -> ("Project Tree"=w260:refnum<vi>)
        n160 = Empty String/Path?(string/path=w256) -> (empty?=w255:bool)
        n161 = case shown="False" w255 {
          tunnel: w260 -> [w271 _]
          tunnel: w259 -> [w267 w272]
          tunnel: [w266 w272] -> w258
          tunnel: w256 -> [w265 _]
          frame False {
            n162 = invoke class="Tree (strict)" method="Open/Close.Ensure Visible"(reference=w271, error in=w267, "tag"=w265) -> (reference out=w270:refnum<vi>, error out=w269:errorcluster)  [unwired: 1 in, 2 out]
            n163 = Build Array(w265) -> (w268:string[])
            n164 = property class="Tree (strict)"(reference=w270, error in=w269, "Val(Sgnl)"=w268) -> (error out=w266:errorcluster)  [unwired: 1 out]
          }
          frame True {
          }
        }
      }
      event "AuditMCLB": Double Click {
        n165 = event-data() -> ("CtlRef"=w283:refnum<vi>, "Row"=w276:i32)  [unwired: 1 in]
        n166 = property class="MCListbox (strict)"(reference=w283) -> ("ItemNames"=w282:string[][])  [unwired: 1 in, 2 out]
        n167 = Unbundle By Name(w280) -> ("Project"=w274:refnum<vi>, "Project Tree"=w279:refnum<vi>)
        n168 = Index Array(array=w282, index (row)=w276, index (col)=0 ("disabled index (col)")) -> (element=w275:string)
        n169 = Empty String/Path?(string/path=w275) -> (empty?=w273:bool)
        n170 = case shown="False" w273 {
          tunnel: w279 -> [w292 _]
          tunnel: w278 -> [w288 w293]
          tunnel: [w286 w293] -> w277
          tunnel: w275 -> [w285 _]
          tunnel: w274 -> [w284 _]
          frame False {
            n171 = invoke class="Tree (strict)" method="Open/Close.Ensure Visible"(reference=w292, error in=w288, "tag"=w285) -> (reference out=w291:refnum<vi>, error out=w290:errorcluster)  [unwired: 1 in, 2 out]
            n172 = Build Array(w285) -> (w289:string[])
            n173 = property class="Tree (strict)"(reference=w291, error in=w290, "Val(Sgnl)"=w289) -> (error out=w287:errorcluster)  [unwired: 1 out]
            n174 = call "VIQA Open File.vi"("error in (no error)"=w287, "Tag"=w285, "Project in"=w284) -> ("error out"=w286:errorcluster)  [unwired: 8 in]
          }
          frame True {
          }
        }
      }
      event Key Down? {
        n175 = event-data() -> ("Char"=w296:i16, "VKey"=w297:T14, "PlatMods"=w301:T13)  [unwired: 1 in, 2 out]
        n176 = Unbundle By Name(w301) -> ("Shift"=w294:bool, "Ctrl"=w300:bool)
        n177 = case shown="True" w300 {
          tunnel: [w303 w307] -> w299
          tunnel: w298 -> [w303 w309]
          tunnel: w297 -> [_ w308]
          tunnel: w296 -> [_ w306]
          tunnel: [_ w305] -> w295
          tunnel: w294 -> [_ w304]
          frame False {
          }
          frame True {
            n178 = case shown="\"Return\"" w308 {
              tunnel: w309 -> [w314 w323 w338 w365 w384]
              tunnel: [w312 w322 w337 w363 w382] -> w307
              tunnel: w306 -> [_ w320 _ _ _]
              tunnel: [w310 w321 w336 w361 w380] -> w305
              tunnel: w304 -> [_ _ w335 _ _]
              frame "Return" {
                n179 = property on="Apply" class="Bool"(error in=w314) -> (error out=w313:errorcluster, "DisabledEnum"=w311:T11)  [unwired: 1 in, 1 out]
                n180 = case shown="\"Enabled\"" w311 {
                  tunnel: w313 -> [w315 w319]
                  tunnel: [w315 w317] -> w312
                  tunnel: [_ TRUE] -> w310
                  frame Default {
                  }
                  frame "Enabled" {
                    n181 = property on="Apply" class="Bool"(error in=w319, "Key Focus"=TRUE) -> (error out=w317:errorcluster)  [unwired: 1 in, 1 out]
                  }
                }
              }
              frame "ASCII", Default {
                n182 = case shown="108" w320 {
                  tunnel: w323 -> [w324 w329]
                  tunnel: [w324 w327] -> w322
                  tunnel: [_ w325] -> w321
                  frame Default {
                  }
                  frame 108 {
                    # "L = Reset Legal Marking"
                    n183 = property on="Reset Legal" class="Bool"(error in=w329) -> (error out=w328:errorcluster, "DisabledEnum"=w326:T11)  [unwired: 1 in, 1 out]
                    n184 = case shown="\"Enabled\"" w326 {
                      tunnel: w328 -> [w330 w334]
                      tunnel: [w330 w332] -> w327
                      tunnel: [_ TRUE] -> w325
                      frame Default {
                      }
                      frame "Enabled" {
                        n185 = property on="Reset Legal" class="Bool"(error in=w334, "Key Focus"=TRUE) -> (error out=w332:errorcluster)  [unwired: 1 in, 1 out]
                      }
                    }
                  }
                }
              }
              frame "Insert" {
                n186 = case shown="False" w335 {
                  tunnel: w338 -> [w343 w354]
                  tunnel: [w341 w352] -> w337
                  tunnel: [w339 w350] -> w336
                  frame False {
                    n187 = property on="VI Description" class="Str"(error in=w343) -> (error out=w342:errorcluster, "DisabledEnum"=w340:T11)  [unwired: 1 in, 1 out]
                    n188 = case shown="\"Enabled\"" w340 {
                      tunnel: w342 -> [w344 w349]
                      tunnel: [w344 w347] -> w341
                      tunnel: [_ TRUE] -> w339
                      frame Default {
                      }
                      frame "Enabled" {
                        n189 = property on="VI Description" class="Str"(error in=w349, "Key Focus"=TRUE, "Text.Selection"=T8 {"Selection Start"=0, "Selection End"=4294967295}) -> (error out=w347:errorcluster)  [unwired: 1 in, 1 out]
                      }
                    }
                  }
                  frame True {
                    n190 = property on="Legal" class="Str"(error in=w354) -> (error out=w353:errorcluster, "DisabledEnum"=w351:T11)  [unwired: 1 in, 1 out]
                    n191 = case shown="\"Enabled\"" w351 {
                      tunnel: w353 -> [w355 w360]
                      tunnel: [w355 w358] -> w352
                      tunnel: [_ TRUE] -> w350
                      frame Default {
                      }
                      frame "Enabled" {
                        n192 = property on="Legal" class="Str"(error in=w360, "Key Focus"=TRUE, "Text.Selection"=T8 {"Selection Start"=0, "Selection End"=4294967295}) -> (error out=w358:errorcluster)  [unwired: 1 in, 1 out]
                      }
                    }
                  }
                }
              }
              frame "PageDown" {
                n193 = property on="AuditMCLB" class="MCListbox (strict)"(error in=w365) -> (error out=w364:errorcluster, "DisabledEnum"=w362:T11)  [unwired: 1 in, 1 out]
                n194 = case shown="Default" w362 {
                  tunnel: w364 -> [w366 w379]
                  tunnel: [w366 w375] -> w363
                  tunnel: [_ TRUE] -> w361
                  frame Default {
                  }
                  frame "Enabled" {
                    n195 = property on="AuditMCLB" class="MCListbox (strict)"(error in=w379, "Key Focus"=TRUE) -> (error out=w376:errorcluster, "Value"=w370:i32, "ItemNames"=w374:string[][])  [unwired: 1 in, 1 out]
                    n196 = Array Size(array=w374) -> (size(s)=w373:i32[])
                    n197 = Index Array(array=w373) -> (element=w372:i32)  [unwired: 1 in]
                    n198 = Decrement(x=w372) -> (x-1=w368:i32)
                    n199 = Greater Or Equal?(x=w370, y=w368) -> (x >= y?=w369:bool)
                    n200 = Increment(x=w370) -> (x+1=w367:i32)
                    n201 = Select(t=w368, s=w369, f=w367) -> (s? t:f=w371:i32)
                    n202 = property on="AuditMCLB" class="MCListbox (strict)"(error in=w376, "Val(Sgnl)"=w371) -> (error out=w375:errorcluster)  [unwired: 1 in, 1 out]
                  }
                }
              }
              frame "PageUp" {
                n203 = property on="AuditMCLB" class="MCListbox (strict)"(error in=w384) -> (error out=w383:errorcluster, "DisabledEnum"=w381:T11)  [unwired: 1 in, 1 out]
                n204 = case shown="\"Enabled\"" w381 {
                  tunnel: w383 -> [w385 w395]
                  tunnel: [w385 w391] -> w382
                  tunnel: [_ TRUE] -> w380
                  frame Default {
                  }
                  frame "Enabled" {
                    n205 = property on="AuditMCLB" class="MCListbox (strict)"(error in=w395, "Key Focus"=TRUE) -> (error out=w392:errorcluster, "Value"=w390:i32)  [unwired: 1 in, 1 out]
                    n206 = Decrement(x=w390) -> (x-1=w388:i32)
                    n207 = Less Or Equal To 0?(x=w390) -> (x <= 0?=w389:bool)
                    n208 = Select(t=0, s=w389, f=w388) -> (s? t:f=w386:i32)
                    n209 = property on="AuditMCLB" class="MCListbox (strict)"(error in=w392, "Val(Sgnl)"=w386) -> (error out=w391:errorcluster)  [unwired: 1 in, 1 out]
                  }
                }
              }
            }
          }
        }
        n210 = event-data("Discard?"=w295) -> ()  [unwired: 1 in, 1 out]
      }
    }
    n211 = call <vilib>:"Simple Error Handler.vi"("error in (no error)"=w34) -> ("error out"=w31:errorcluster)  [unwired: 4 in, 4 out]
    n212 = call <vilib>:"Clear Errors.vi"("error in (no error)"=w31) -> ("error out"=w30:errorcluster)  [unwired: 5 in, 1 out]
  }
  n213 = Unbundle By Name(w23) -> ("Abort"=w3:refnum<vi>, "AuditMCLB"=w9:refnum<vi>, "AuditSlide"=w10:refnum<vi>, "Project Tree"=w19:refnum<vi>, "App Ref"=w16:refnum<vi>, "Project"=w20:refnum<vi>, "My Computer"=w21:refnum<vi>, "VI Refnum"=w22:refnum<vi>)
  n214 = Close Reference(reference=w22) -> ()  [unwired: 1 in, 1 out]
  n215 = Close Reference(reference=w21) -> ()  [unwired: 1 in, 1 out]
  n216 = Close Reference(reference=w20) -> ()  [unwired: 1 in, 1 out]
  n217 = Close Reference(reference=w16) -> ()  [unwired: 1 in, 1 out]
  n218 = Close Reference(reference=w19) -> ()  [unwired: 1 in, 1 out]
  n219 = Close Reference(reference=w10) -> ()  [unwired: 1 in, 1 out]
  n220 = Close Reference(reference=w9) -> ()  [unwired: 1 in, 1 out]
  n221 = Close Reference(reference=w3) -> ()  [unwired: 1 in, 1 out]
